vi "Demodulation (SubVI).vi"(0 "pilot_offset_time":i16, 1 "pilot_offset_freq":i16, 2 "frame_length":i64, 5 "H_est":cdb[](array[numeric]), 7 "SC_total":i16, 9 "OFDM_output":cdb[][](array[numeric]), 12 "SC_pilot":i16, 13 "SC_data":i64, 14 "est_ploc_mtx":i32[](array[numeric])) -> (4 "demod_data":i8[](array[numeric]))   [LabVIEW 2015]
uses:
  <vilib>/imath/engines/lvmath2/RunTimeEngine/RangeToken/NIMS_Range.vi
  <instcachedir>/0/NIMS_Range_D919CC09935940E88F755EC1C6F49AC1.lvgen/NIMS_Range_D919CC09935940E88F755EC1C6F49AC1_001.vi
  <instcachedir>/0/NIMS_Range_D919CC09935940E88F755EC1C6F49AC1.lvgen/NIMS_Range_D919CC09935940E88F755EC1C6F49AC1_000.vi
  <vilib>/imath/engines/lvmath2/RunTimeSupport/NIMS_Error if Not Equal.vi
  <instcachedir>/0/NIMS_Error if Not Equal_7F0D61CE56BF44979916ECA34C78675F.lvgen/NIMS_Error if Not Equal_7F0D61CE56BF44979916ECA34C78675F_001.vi
  <vilib>/imath/engines/lvmath2/RunTimeEngine/IndexRead/NIMS V(V).vi
  <instcachedir>/0/NIMS V(V)_298D9CB7BFEB42B8BC8D9C3C28AE8C70.lvgen/NIMS V(V)_298D9CB7BFEB42B8BC8D9C3C28AE8C70_000.vi
  <vilib>/imath/engines/lvmath2/RunTimeEngine/BuiltInFunctions/sets_diff/NIMS_sets_diff(GV2).vi
  <instcachedir>/0/NIMS_sets_diff(GV2)_CE188B9DAFCC49368CD9C62F83DF72AA.lvgen/NIMS_sets_diff(GV2)_CE188B9DAFCC49368CD9C62F83DF72AA_007.vi
  <vilib>/imath/engines/lvmath2/RunTimeEngine/ErrorHandling/NIMS_Create Error From Enums.vi
  <vilib>/imath/engines/lvmath2/RunTimeEngine/IndexRead/NIMS V(R2).vi
  <instcachedir>/0/NIMS V(R2)_C76619605A0E4E9F8B2FA9389712AC47.lvgen/NIMS V(R2)_C76619605A0E4E9F8B2FA9389712AC47_002.vi
  <vilib>/imathl/engines/lvmath/Functions/Error Handling/Create Error.vi
  <instcachedir>/0/NIMS V(V)_298D9CB7BFEB42B8BC8D9C3C28AE8C70.lvgen/NIMS V(V)_298D9CB7BFEB42B8BC8D9C3C28AE8C70_001.vi
  <vilib>/imath/engines/lvmath2/RunTimeEngine/IndexRead/NIMS M($,V).vi
  <instcachedir>/0/NIMS M($,V)_706F2CE2C8E141269FD4C8A402E169C5.lvgen/NIMS M($,V)_706F2CE2C8E141269FD4C8A402E169C5_000.vi
  <vilib>/imath/engines/lvmath2/RunTimeEngine/BuiltInFunctions/length/NIMS_length(GV).vi
  <instcachedir>/0/NIMS_length(GV)_08A3D13377FD4E4B96F5795FBF3698FA.lvgen/NIMS_length(GV)_08A3D13377FD4E4B96F5795FBF3698FA_002.vi
  <vilib>/imath/engines/lvmath2/RunTimeEngine/RangeToken/NIMS_Range_R2 - Integer.vi
  <instcachedir>/0/NIMS_Range_R2 - Integer_396D5D4FB869421F9245109A0975AD54.lvgen/NIMS_Range_R2 - Integer_396D5D4FB869421F9245109A0975AD54_000.vi
  <vilib>/imath/engines/lvmath2/RunTimeEngine/CommandStatement/MC_CommandStatement_break.vi
  <instcachedir>/0/NIMS_length(GV)_08A3D13377FD4E4B96F5795FBF3698FA.lvgen/NIMS_length(GV)_08A3D13377FD4E4B96F5795FBF3698FA_001.vi
  <vilib>/imath/engines/lvmath2/RunTimeEngine/BuiltInFunctions/zeros/NIMS_V=zeros(I32,I32).vi
  <vilib>/imath/engines/lvmath2/RunTimeEngine/IndexRead/NIMS M(S,S).vi
  <instcachedir>/0/NIMS M(S,S)_AC51E74150A542F7991B9634C66F3096.lvgen/NIMS M(S,S)_AC51E74150A542F7991B9634C66F3096_001.vi
  <vilib>/imath/engines/lvmath2/RunTimeEngine/IndexRead/NIMS V(S).vi
  <instcachedir>/0/NIMS V(S)_0488751826AF41519A22953C041130DC.lvgen/NIMS V(S)_0488751826AF41519A22953C041130DC_003.vi
  <vilib>/imath/engines/lvmath2/RunTimeEngine/BuiltInFunctions/abs/NIMS_abs(signed).vi
  <instcachedir>/0/NIMS_abs(signed)_C4FCB8E6058B49B797C7C8D53CA5F6EC.lvgen/NIMS_abs(signed)_C4FCB8E6058B49B797C7C8D53CA5F6EC_002.vi
  <vilib>/imath/engines/lvmath2/RunTimeEngine/IndexReplace/NIMS V(S)=S.vi
  <instcachedir>/0/NIMS V(S)=S_9916D32195284AEB9D40BA9A64F3B0C5.lvgen/NIMS V(S)=S_9916D32195284AEB9D40BA9A64F3B0C5_000.vi
  <vilib>/imath/engines/lvmath2/RunTimeEngine/BuiltInFunctions/min/1 input/NIMS_min(RV).vi
  <instcachedir>/0/NIMS_min(RV)_EE2DD3E2888846108C5160A664B67832.lvgen/NIMS_min(RV)_EE2DD3E2888846108C5160A664B67832_000.vi
  <vilib>/imath/engines/lvmath2/RunTimeEngine/VariableToken/NIMS_VariableToken_CondDefinedDefinedByReplace.vi
  <instcachedir>/0/NIMS_VariableToken_CondDefinedDefinedByReplace_D162CFFC24174562A9FEA619A91E1A56.lvgen/NIMS_VariableToken_CondDefinedDefinedByReplace_D162CFFC24174562A9FEA619A91E1A56_002.vi
  <vilib>/imath/engines/lvmath2/RunTimeEngine/IndexReplace/NIMS V(R2)=V.vi
  <instcachedir>/0/NIMS V(R2)=V_A4A1DC5DDA874862BD08E3229D1DC268.lvgen/NIMS V(R2)=V_A4A1DC5DDA874862BD08E3229D1DC268_000.vi
  <vilib>/imath/engines/lvmath2/RunTimeEngine/VariableToken/NIMS_VariableToken_CondDefined.vi
  <instcachedir>/0/NIMS_VariableToken_CondDefined_FE30D0A1BFB24F098D41DEBABFE96BE1.lvgen/NIMS_VariableToken_CondDefined_FE30D0A1BFB24F098D41DEBABFE96BE1_003.vi
  <vilib>/imath/engines/lvmath2/RunTimeEngine/NodeEndStatement/NIMS_NodeEndStatement_Output.vi
  <instcachedir>/0/NIMS_NodeEndStatement_Output_53EC0D466D134D7ABD903AC30B43404B.lvgen/NIMS_NodeEndStatement_Output_53EC0D466D134D7ABD903AC30B43404B_004.vi
  <vilib>/imath/engines/lvmath2/RunTimeEngine/ErrorHandling/NIMS_Finalize Error.vi
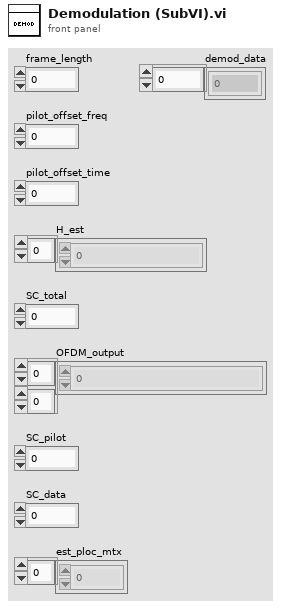
[diagram p1: front panel]
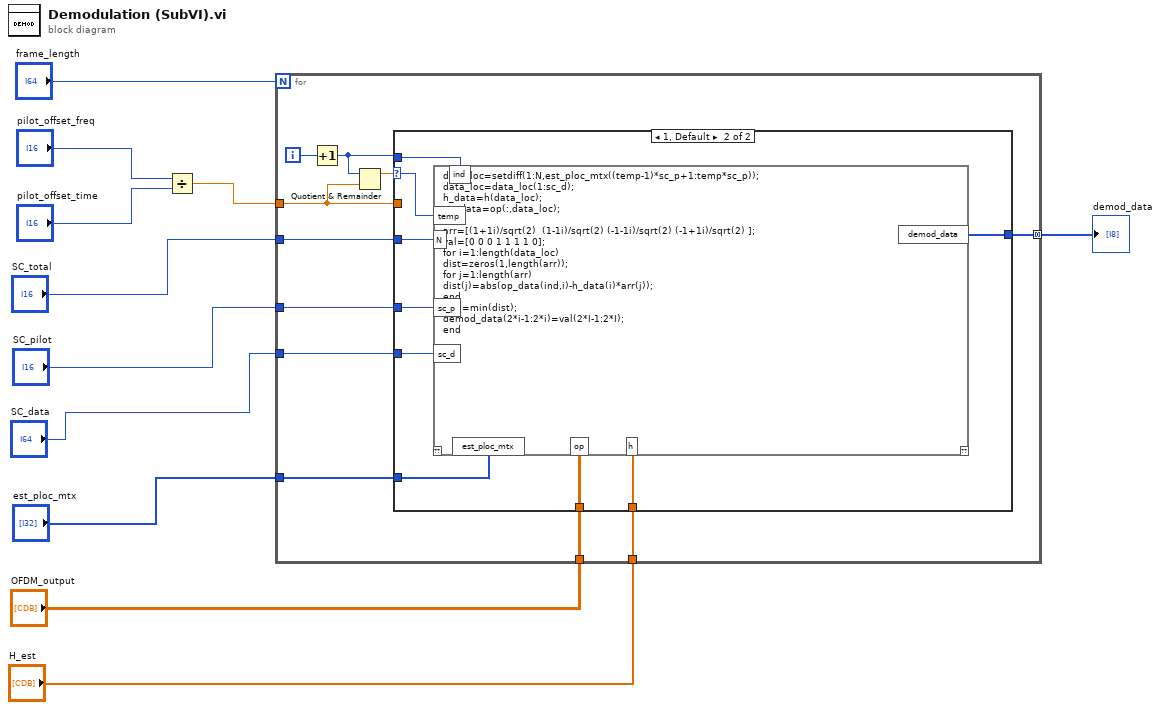
[diagram p0: block diagram]
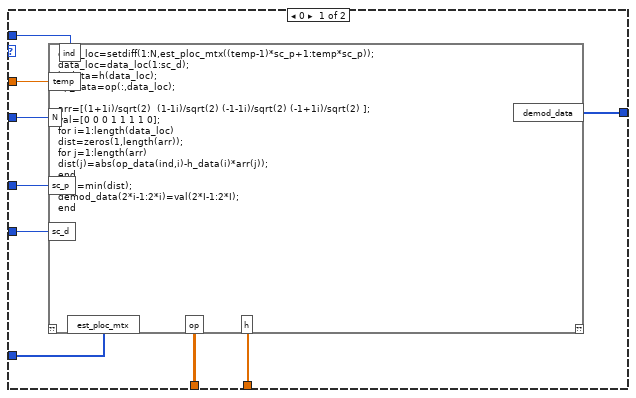
[diagram p2: hidden frame]
diagram:
  n1 = Divide(x="pilot_offset_freq", y="pilot_offset_time") -> (x/y=w2:dbl)
  n2 = for {
    N: "frame_length" -> [_]
    tunnel: w2 -> [w14]
    tunnel: "est_ploc_mtx" -> [w21]
    tunnel: "SC_total" -> [w20]
    tunnel: "SC_pilot" -> [w19]
    tunnel: "SC_data" -> [w18]
    tunnel: "OFDM_output" -> [w17]
    tunnel: "H_est" -> [w16]
    tunnel: [w15] -> w11 mode=concatenating
    i -> [w13]
    n3 = Increment(x=w13) -> (x+1=w12:i32)
    n4 = Quotient & Remainder(x=w12, y=w14) -> (x-y*floor(x/y)=w22:dbl)  [unwired: 1 out]
    n5 = case shown="1, Default" w22 {
      selector: w22 -> [_ w428]
      tunnel: w21 -> [w28 w429]
      tunnel: w20 -> [w31 w430]
      tunnel: w19 -> [w30 w427]
      tunnel: w18 -> [w29 w426]
      tunnel: w17 -> [w27 w425]
      tunnel: w16 -> [w26 w424]
      tunnel: [w25 w423] -> w15
      tunnel: w14 -> [w24 _]
      tunnel: w12 -> [w23 w422]
      frame 0 {
        n6 = mathscript code="data_loc=setdiff(1:N,est_ploc_mtx((temp-1)*sc_p+1:temp*sc_p));\ndata_loc=data_loc(1:sc_d);\nh_data=h(data_loc);\nop_data=op(:,data_loc);\n\narr=[(1+1i)/sqrt(2)  (1-1i)/sqrt(2) (-1-1i)/sqrt(2) (-1+1i)/sqrt(2) ];\nval=[0 0 0 1 1 1 1 0];\nfor i=1:length(data_loc)\ndist=zeros(1,length(arr));\nfor j=1:length(arr)\ndist(j)=abs(op_data(ind,i)-h_data(i)*arr(j));\nend\n[x,I]=min(dist);\ndemod_data(2*i-1:2*i)=val(2*I-1:2*I);\nend"("est_ploc_mtx"=w28, "N"=w31, "temp"=w24, "sc_p"=w30, "sc_d"=w29, "op"=w27, "h"=w26, "ind"=w23) -> ("demod_data"=w25:i32[])  [unwired: 1 in, 1 out]
      }
      frame 1, Default {
        n7 = mathscript code="data_loc=setdiff(1:N,est_ploc_mtx((temp-1)*sc_p+1:temp*sc_p));\ndata_loc=data_loc(1:sc_d);\nh_data=h(data_loc);\nop_data=op(:,data_loc);\n\narr=[(1+1i)/sqrt(2)  (1-1i)/sqrt(2) (-1-1i)/sqrt(2) (-1+1i)/sqrt(2) ];\nval=[0 0 0 1 1 1 1 0];\nfor i=1:length(data_loc)\ndist=zeros(1,length(arr));\nfor j=1:length(arr)\ndist(j)=abs(op_data(ind,i)-h_data(i)*arr(j));\nend\n[x,I]=min(dist);\ndemod_data(2*i-1:2*i)=val(2*I-1:2*I);\nend"("est_ploc_mtx"=w429, "N"=w430, "temp"=w428, "sc_p"=w427, "sc_d"=w426, "op"=w425, "h"=w424, "ind"=w422) -> ("demod_data"=w423:i32[])  [unwired: 1 in, 1 out]
      }
    }
  }
  "demod_data" <- w11
